vi "posi inicial- proceso 2.vi"() -> ()   [LabVIEW 2020]
panel:
  out "posi-inicial proceso 2":T1
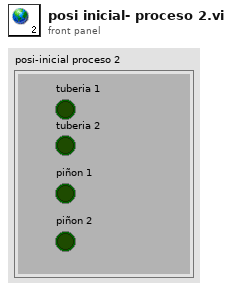
[diagram p1: front panel]
types:
  T1 = cluster{"tuberia 1":bool, "tuberia 2":bool, "piñon 1":bool, "piñon 2":bool}
diagram:
